vi "XYZ to NormXYZ.vi"(0 "X start":dbl, 1 "Y start":dbl, 3 "X stop":dbl, 4 "Y stop":dbl, 5 "Zoom (either ref or main zoom)":dbl, 6 "FrameSize":i32, 7 "Z start":dbl, 9 "Z stop":dbl) -> (14 "Norm X Start":dbl, 15 "Norm Y Start":dbl, 16 "Norm Z Start":dbl, 17 "Norm X Stop":dbl, 18 "Norm Y Stop":dbl, 19 "Norm Z Stop":dbl)   [LabVIEW 2020]
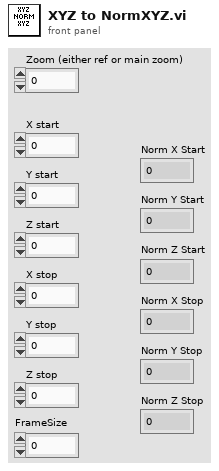
[diagram p1: front panel]
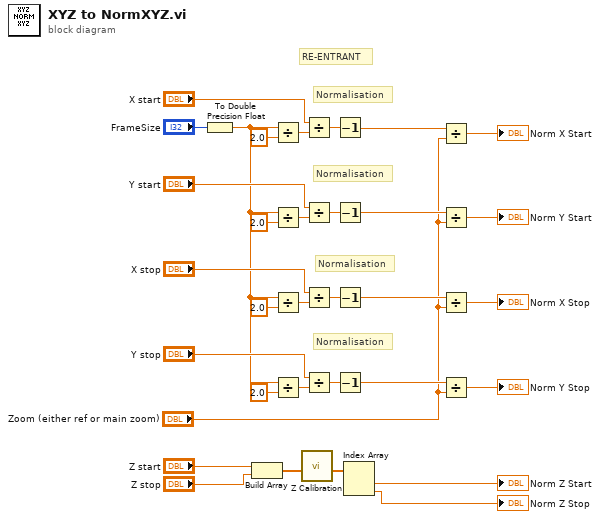
[diagram p0: block diagram]
diagram:
  # "RE-ENTRANT"
  # "Normalisation"
  # "Normalisation"
  # "Normalisation"
  # "Normalisation"
  n1 = To Double Precision Float(number="FrameSize") -> (double precision float=w16:dbl)
  n2 = Build Array("Z start", "Z stop") -> (w4:dbl[])
  n3 = Divide(x=w16, y=2.0) -> (x/y=w28:dbl)
  n4 = Divide(x=w16, y=2.0) -> (x/y=w25:dbl)
  n5 = Divide(x=w16, y=2.0) -> (x/y=w23:dbl)
  n6 = Divide(x=w16, y=2.0) -> (x/y=w19:dbl)
  n7 = call "Z Calibration.vi"("Z Planes"=w4) -> ("Norm Z"=w3:dbl[])  [unwired: 7 in, 3 out]
  n8 = Divide(x="X start", y=w28) -> (x/y=w17:dbl)
  n9 = Divide(x="Y start", y=w25) -> (x/y=w24:dbl)
  n10 = Divide(x="X stop", y=w23) -> (x/y=w21:dbl)
  n11 = Divide(x="Y stop", y=w19) -> (x/y=w18:dbl)
  n12 = Decrement(x=w17) -> (x-1=w11:dbl)
  n13 = Decrement(x=w24) -> (x-1=w13:dbl)
  n14 = Decrement(x=w21) -> (x-1=w15:dbl)
  n15 = Decrement(x=w18) -> (x-1=w14:dbl)
  n16 = Index Array(array=w3) -> (element #1=→"Norm Z Start":dbl, element #2=→"Norm Z Stop":dbl)  [unwired: 2 in]
  n17 = Divide(x=w11, y="Zoom (either ref or main zoom)") -> (x/y=→"Norm X Start":dbl)
  n18 = Divide(x=w13, y="Zoom (either ref or main zoom)") -> (x/y=→"Norm Y Start":dbl)
  n19 = Divide(x=w15, y="Zoom (either ref or main zoom)") -> (x/y=→"Norm X Stop":dbl)
  n20 = Divide(x=w14, y="Zoom (either ref or main zoom)") -> (x/y=→"Norm Y Stop":dbl)
